vi "test Message - Clear.vi"(8 "error in (no error)":errorcluster, 11 "TestCase in":refnum<class "Test_Queue.lvclass">) -> (0 "error out":errorcluster, 3 "TestCase out":refnum<class "Test_Queue.lvclass">)   [LabVIEW 2015, in "Test_Queue.lvclass"]
uses:
  Test_Queue.lvclass
  Global Parameters.vi
  Core/Session/Session.lvclass
  Queue/NI_Azure_Queue.lvlib
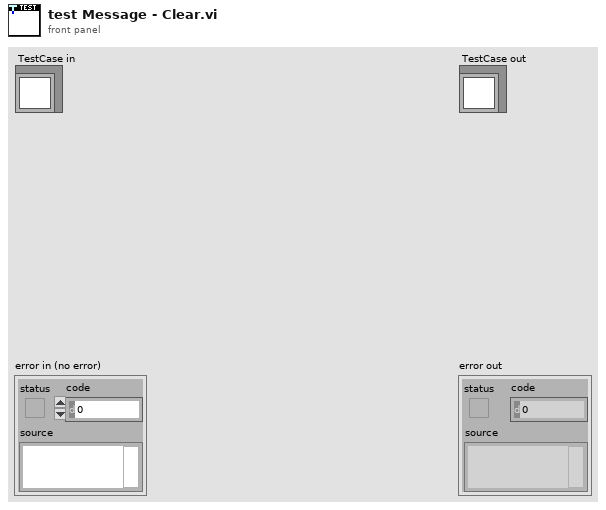
[diagram p1: front panel]
types:
  T1 = typedef "NI_Azure_Core.lvlib/Azure Credentials.ctl" = cluster{"Storage Account Name":string, "Access Key":string}
  T2 = typedef "NI_Azure_Queue.lvlib/Message.ctl" = cluster{"Message ID":string, "Insertion Time":string, "Expiration Time":string, "Pop Receipt":string, "Time Next Visible":string, "Dequeue Count":i32, "Message Text":string}
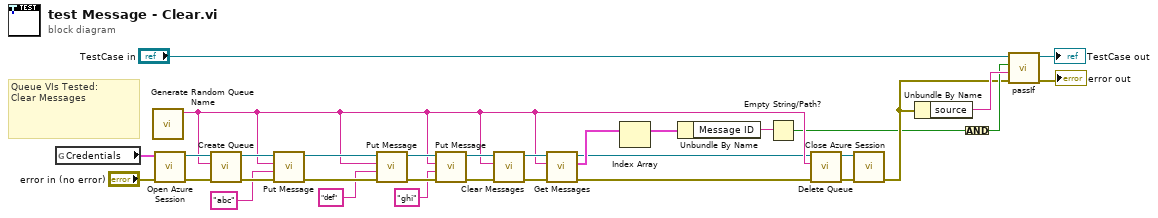
[diagram p0: block diagram]
diagram:
  # "Queue VIs Tested:\nClear Messages"
  n1 = global read "Global Parameters.vi" "Credentials"() -> (w26:T1)
  n2 = call "Generate Random Queue Name.vi"() -> ("Random Queue Name"=w6:string)  [unwired: 11 in]
  n3 = call "Open Azure Session.vi"("error in (no error)"="error in (no error)", "Credentials"=w26) -> ("error out"=w27:errorcluster, "Azure Session"=w22:refnum<class "Session.lvclass">)  [unwired: 8 in]
  n4 = call "Create Queue.vi"("error in (no error)"=w27, "Queue"=w6, "Azure Session in"=w22) -> ("error out"=w23:errorcluster, "Azure Session out"=w18:refnum<class "Session.lvclass">)  [unwired: 7 in]
  n5 = call "Put Message.vi"("error in (no error)"=w23, "Message"="abc", "Queue"=w6, "Azure Session in"=w18) -> ("error out"=w19:errorcluster, "Azure Session out"=w17:refnum<class "Session.lvclass">)  [unwired: 5 in, 1 out]
  n6 = call "Put Message.vi"("error in (no error)"=w19, "Message"="def", "Queue"=w6, "Azure Session in"=w17) -> ("error out"=w14:errorcluster, "Azure Session out"=w13:refnum<class "Session.lvclass">)  [unwired: 5 in, 1 out]
  n7 = call "Put Message.vi"("error in (no error)"=w14, "Message"="ghi", "Queue"=w6, "Azure Session in"=w13) -> ("error out"=w11:errorcluster, "Azure Session out"=w10:refnum<class "Session.lvclass">)  [unwired: 5 in, 1 out]
  n8 = call "Clear Messages.vi"("error in (no error)"=w11, "Queue"=w6, "Azure Session in"=w10) -> ("error out"=w9:errorcluster, "Azure Session out"=w8:refnum<class "Session.lvclass">)  [unwired: 7 in]
  n9 = call "Get Messages.vi"("error in (no error)"=w9, "Queue"=w6, "Azure Session in"=w8) -> ("error out"=w7:errorcluster, "Messages"=w4:T2[], "Azure Session out"=w3:refnum<class "Session.lvclass">)  [unwired: 6 in]
  n10 = Index Array(array=w4) -> (element=w1:T2)  [unwired: 1 in]
  n11 = Unbundle By Name(w1) -> ("Message ID"=w5:string)
  n12 = Empty String/Path?(string/path=w5) -> (empty?=w2:bool)
  n13 = call "Delete Queue.vi"("error in (no error)"=w7, "Queue"=w6, "Azure Session in"=w3) -> ("error out"=w21:errorcluster, "Azure Session out"=w20:refnum<class "Session.lvclass">)  [unwired: 7 in]
  n14 = call "Close Azure Session.vi"("error in (no error)"=w21, "Azure Session"=w20) -> ("error out"=w24:errorcluster)  [unwired: 9 in]
  n15 = Unbundle By Name(w24) -> ("source"=w29:string)
  n16 = Compound Arithmetic op=AND(w2) -> (w25:bool)
  n17 = call-dynamic "passIf.vi"("error in (no error)"=w24, "message (\"\")"=w29, "pass"=w25, "TestCase in"="TestCase in") -> ("error out"=→"error out":errorcluster, "TestCase out"=→"TestCase out":refnum<class "Test_Queue.lvclass">)  [unwired: 6 in]
